vi "Teleop.vi"(10 "Match Info":T1={"Autonomous Elapsed Seconds"=0.0, "TeleOp Elapsed Seconds"=0.0, "Disabled Elapsed Seconds"=0.0, "Visited Autonomous"=FALSE, "Visited TeleOp"=FALSE, "Visited Disabled"=FALSE, "Autonomous Settings"={"Autonomous Style"=enum."Independent", "VI Refnum"=refnum}}, 11 "Call Context":T2) -> ()   [LabVIEW 2016]
doc: "This VI is called for each TeleOp packet received from the DS where the robot is not disabled. It is often used to read from the joysticks and update I/O or to update setpoints for timed control loops. It should complete and return within 20 milliseconds or it may miss DS packets."
uses:
  <vilib>/Rock Robotics/WPI/DriverStation/WPI_DriverStationDerivedRobotMode.ctl
  <vilib>/Rock Robotics/WPI/DriverStation/WPI_DriverStationMatch Info.ctl
  <vilib>/Rock Robotics/WPI/Utilities/WPI_GetSetVariantRefNum.vi
  Robot Global Data.vi
  <vilib>/Rock Robotics/Network Tables/NT Write Boolean Array.vi
  <vilib>/Rock Robotics/Network Tables/NT Write Numeric Array.vi
  <vilib>/Rock Robotics/Network Tables/NT Read Boolean.vi
  <vilib>/Rock Robotics/Network Tables/NT Read Number.vi
  <vilib>/Rock Robotics/WPI/Ultrasonic/WPI_SonarMB1010AnalogRefNum Registry Get.vi
  <vilib>/Rock Robotics/WPI/Ultrasonic/WPI_SonarMB1010AnalogGetRange.vi
  <vilib>/Rock Robotics/Network Tables/NT Write Boolean.vi
  <vilib>/Rock Robotics/Network Tables/NT Write Number.vi
  <vilib>/Rock Robotics/WPI/RobotDrive/WPI_RobotDriveMecanumDrive_Cartesian.vi
panel:
  out "Sample Slider 0":dbl(slide) scale=0.0..5.0
  out "Sample Boolean 1":bool
  out "Sample Boolean 0":bool
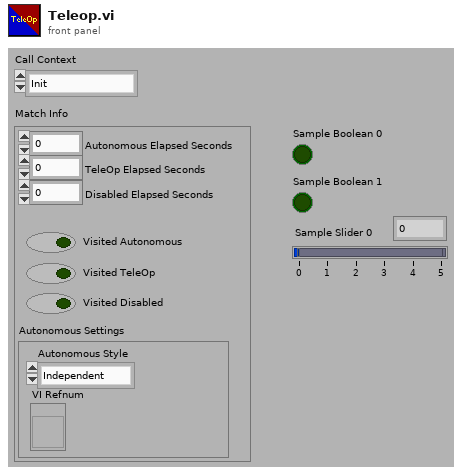
[diagram p1: front panel]
types:
  T1 = typedef "WPI_DriverStationMatch Info.ctl" = cluster{"Autonomous Elapsed Seconds":dbl, "TeleOp Elapsed Seconds":dbl, "Disabled Elapsed Seconds":dbl, "Visited Autonomous":bool, "Visited TeleOp":bool, "Visited Disabled":bool, "Autonomous Settings":cluster{"Autonomous Style":enum16{"Iterative", "Independent"}, "VI Refnum":refnum<vi>}}
  T2 = typedef "WPI_DriverStationDerivedRobotMode.ctl" = enum16{"Init", "Execute", "Stop"}
  T3 = typedef "WPI_JoystickDevRef.ctl" = cluster{"Device":T4}
  T4 = typedef "WPI_JoystickDeviceEnum.ctl" = enum16{"USB 0", "USB 1", "USB 2", "USB 3", "USB 4", "USB 5"}
  T5 = typedef "WPI_RobotDriveDevRef.ctl" = cluster{"DevStatus":errorcluster, "Motors[]":T6[], "Square Inputs":bool, "Max Output":dbl}
  T6 = typedef "WPI_MotorControlDeviceRef.ctl" = cluster{"DeviceStatus":errorcluster, "Type":T7, "PWM":cluster{"PWM Channel":T8, "DeadBand":T9}, "CAN":cluster{"Device Number":u8, "SetOutput VI Ref":variant, "GetOutput VI Ref":variant, "Enable VI Ref":variant, "Disable VI Ref":variant, "Data":variant}, "Invert":bool}
  T7 = typedef "WPI_MotorControlType.ctl" = enum16{"PWM", "CAN"}
  T8 = typedef "FPGA_DIOPWMChannel.ctl" = enum8{"PWM 0", "PWM 1", "PWM 2", "PWM 3", "PWM 4", "PWM 5", "PWM 6", "PWM 7", "PWM 8", "PWM 9", "PWM MXP 0", "PWM MXP 1", "PWM MXP 2", "PWM MXP 3", "PWM MXP 4", "PWM MXP 5", "PWM MXP 6", "PWM MXP 7", "PWM MXP 8", "PWM MXP 9", "Invalid"}
  T9 = typedef "WPI_PWMDeadband.ctl" = cluster{"Name":string, "maxPositivePwm":i32, "minPositivePwm":i32, "centerPwm":i32, "maxNegativePwm":i32, "minNegativePwm":i32, "angularRange":u16}
  T10 = typedef "WPI_ServoDeviceRef.ctl" = cluster{"DeviceStatus":errorcluster, "PWM Channel":T8, "DeadBand":T9}
  T11 = cluster{"Buttons[0]":bool, "Buttons[1]":bool, "Buttons[2]":bool, "Buttons[3]":bool, "Buttons[4]":bool, "Buttons[5]":bool, "Buttons[6]":bool, "Buttons[7]":bool, "Buttons[8]":bool}
  T12 = typedef "WPI_SwitchDevRef.ctl" = cluster{"DevStatus":errorcluster, "DIO Channel":T13, "CntIndex":T14, "Normally Closed":bool}
  T13 = typedef "FPGA_DIOChannel.ctl" = enum8{"DIO 0", "DIO 1", "DIO 2", "DIO 3", "DIO 4", "DIO 5", "DIO 6", "DIO 7", "DIO 8", "DIO 9", "DIO MXP 0", "DIO MXP 1", "DIO MXP 2", "DIO MXP 3", "DIO MXP 4", "DIO MXP 5", "DIO MXP 6", "DIO MXP 7", "DIO MXP 8", "DIO MXP 9", "DIO MXP 10", "DIO MXP 11", "DIO MXP 12", "DIO MXP 13", "DIO MXP 14", "DIO MXP 15", "SPI Port CS1", "SPI Port CS2", "SPI Port CS3", "SPI Port MISO", "SPI Port MOSI", "Invalid"}
  T14 = typedef "FPGA_CounterCtrSystemIndex.ctl" = enum8{"Ctr 0", "Ctr 1", "Ctr 2", "Ctr 3", "Ctr 4", "Ctr 5", "Ctr 6", "Ctr 7", "Invalid"}
  T15 = typedef "WPI_SonarMB1010AnalogDeviceRef.ctl" = cluster{"AIDeviceRef":T16, "Scaling factor (V/in)":dbl, "Average Bits":u8}
  T16 = typedef "WPI_AnalogChannelDevRef.ctl" = cluster{"DevStatus":errorcluster, "Analog Channel":T17}
  T17 = typedef "FPGA_AIChannel.ctl" = enum8{"AI 0", "AI 1", "AI 2", "AI 3", "AI MXP 0", "AI MXP 1", "AI MXP 2", "AI MXP 3", "Invalid"}
  T18 = typedef "WPI_DigitalInputDevRef.ctl" = cluster{"DevStatus":errorcluster, "DIO Channel":T13}
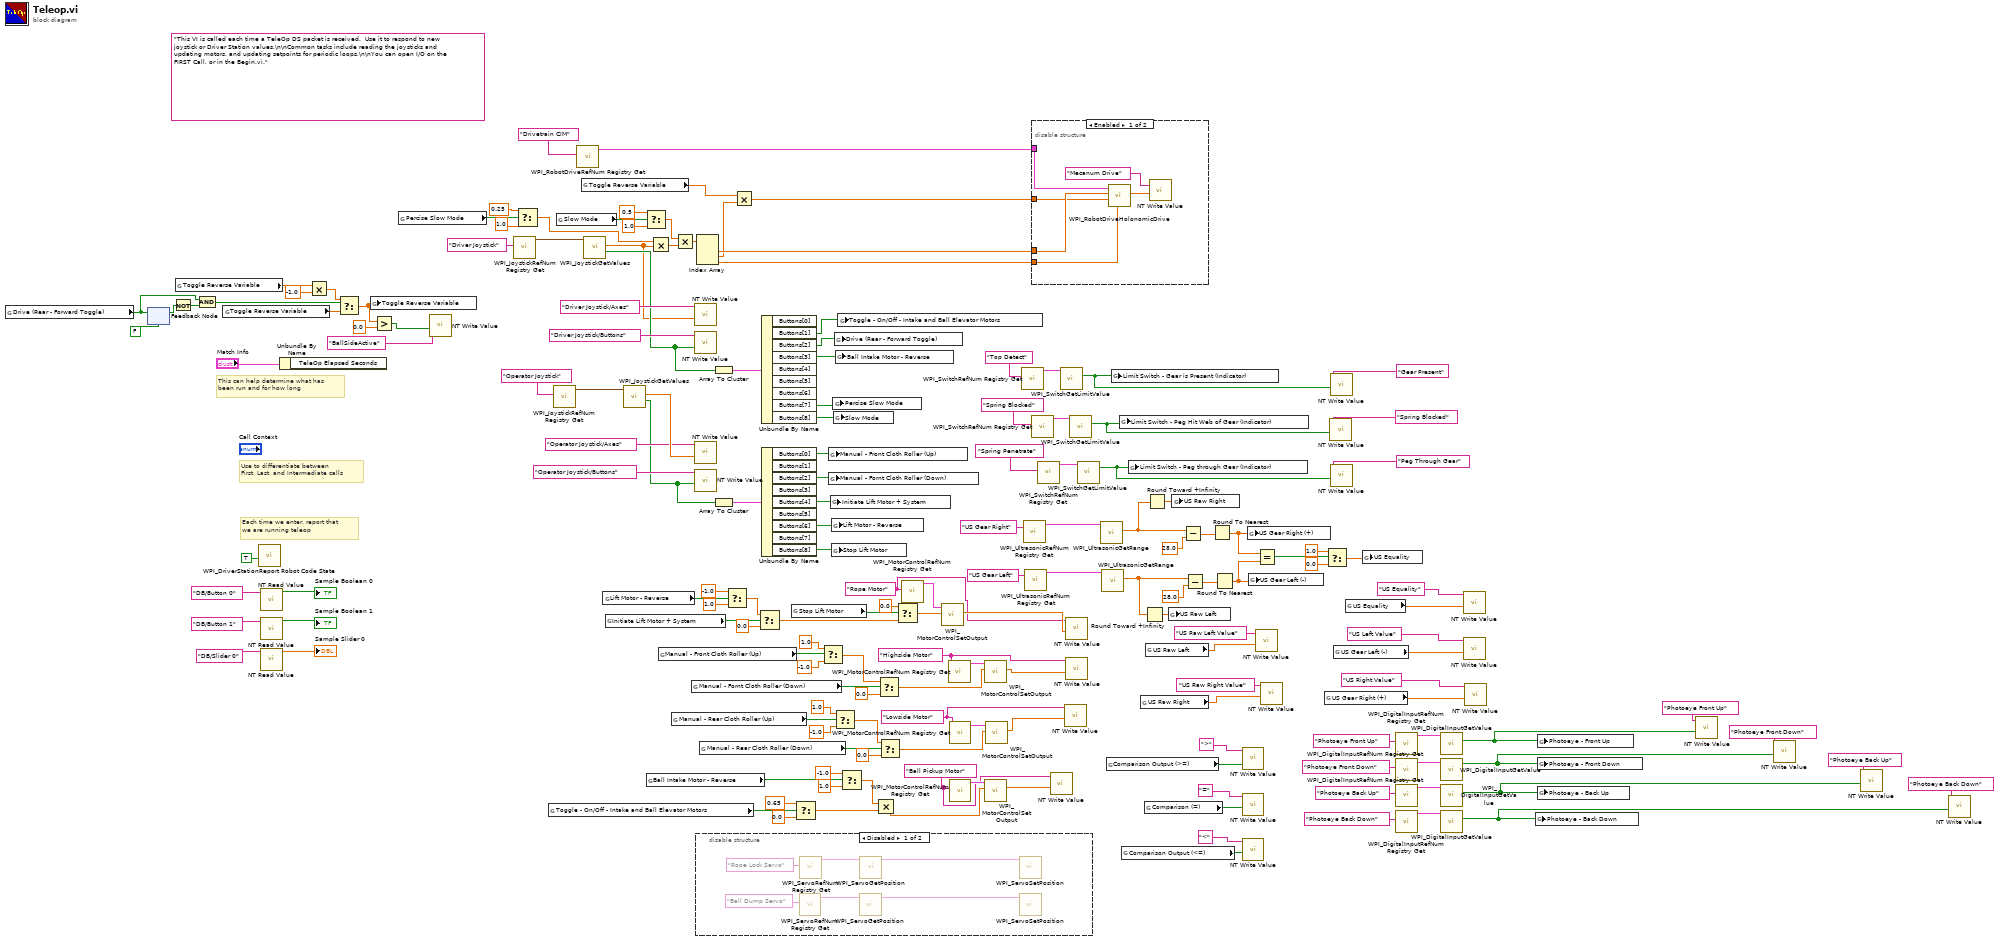
[diagram p0: block diagram]
diagram:
  w5 = "Ball Pickup Motor" ("refnum name")
  w6 = "Lowside Motor" ("refnum name")
  w7 = "Highside Motor" ("refnum name")
  w11 = "Rope Motor" ("refnum name")
  (unwired) "This VI is called each time a TeleOp DS packet is received.  Use it to respond to new joystick or Driver Station values.\n\nCommon tasks include reading the joysticks and updating motors, and updating setpoints for periodic loops.\n\nYou can open I/O on the FIRST Call, or in the Begin.vi."
  # "Each time we enter, report that\nwe are running teleop"
  # "Use to differentiate between\nFirst, Last, and Intermediate calls"
  # "This can help determine what has\nbeen run and for how long"
  n1 = global read "Robot Global Data.vi" "Drive (Rear - Forward Toggle)"() -> (w25:bool)
  n2 = feedback #1(FALSE ("Comparison Output (<=)")) -> (w27:bool)
  n3 = feedback-in #1(w25) -> ()
  n4 = Not(x=w27) -> (.not. x?=w26:bool)
  n5 = global read "Robot Global Data.vi" "Toggle Reverse Variable"() -> (w22:dbl)
  n6 = And(x=w25, y=w26) -> (x .and. y?=w24:bool)
  n7 = global read "Robot Global Data.vi" "Toggle Reverse Variable"() -> (w23:dbl)
  n8 = call <vilib>:"WPI_DriverStationReport Robot Code State.vi"("TeleOp"=TRUE ("Autonomous")) -> ()  [unwired: 10 in, 1 out]
  n9 = call-poly <vilib>:"NT Read Value.vi"("Name"="DB/Button 0" ("refnum name")) -> ("Boolean"=→"Sample Boolean 0":bool)  [unwired: 9 in, 1 out]
  n10 = call-poly <vilib>:"NT Read Value.vi"("Name"="DB/Button 1" ("refnum name")) -> ("Boolean"=→"Sample Boolean 1":bool)  [unwired: 9 in, 1 out]
  n11 = call-poly <vilib>:"NT Read Value.vi"("Name"="DB/Slider 0" ("refnum name")) -> ("Numeric"=→"Sample Slider 0":dbl)  [unwired: 9 in, 1 out]
  n12 = Unbundle By Name("Match Info") -> ()  [unwired: 1 out]
  n13 = Multiply(x=w22, y=-1.0) -> (x*y=w20:dbl)
  n14 = Select(t=w20, s=w24, f=w23) -> (s? t:f=w4:dbl)
  n15 = global write "Robot Global Data.vi" "Toggle Reverse Variable"(w4) -> ()
  n16 = Greater?(x=w4, y=0.0) -> (0:w2:bool)
  n17 = global read "Robot Global Data.vi" "Percise Slow Mode"() -> (w72:bool)
  n18 = call-poly <vilib>:"NT Write Value.vi"("Boolean"=w2, "Name"="BallSideActive") -> ()  [unwired: 9 in, 1 out]
  n19 = call <vilib>:"WPI_JoystickRefNum Registry Get.vi"("refnum name"="Driver Joystick") -> ("JoystickDevRef"=w165:T3)  [unwired: 1 in, 9 out]
  n20 = Select(t=0.25, s=w72, f=1.0) -> (s? t:f=w73:dbl)
  n21 = global read "Robot Global Data.vi" "Toggle - On/Off - Intake and Ball Elevator Motors"() -> (w80:bool)
  n22 = call <vilib>:"WPI_JoystickRefNum Registry Get.vi"("refnum name"="Operator Joystick") -> ("JoystickDevRef"=w147:T3)  [unwired: 9 in, 1 out]
  n23 = global read "Robot Global Data.vi" "Slow Mode"() -> (w151:bool)
  n24 = call <vilib>:"WPI_RobotDriveRefNum Registry Get.vi"("refnum name"="Drivetrain CIM") -> ("RobotDriveDevRef"=w167:T5)  [unwired: 1 in, 9 out]
  n25 = global read "Robot Global Data.vi" "Toggle Reverse Variable"() -> (w17:dbl)
  n26 = call <vilib>:"WPI_JoystickGetValues.vi"("JoystickDevRef"=w165) -> ("Buttons"=w150:bool[], "Axes"=w75:dbl[])  [unwired: 6 in, 3 out]
  n27 = global read "Robot Global Data.vi" "Lift Motor - Reverse"() -> (w103:bool)
  n28 = global read "Robot Global Data.vi" "Initiate Lift Motor + System"() -> (w104:bool)
  n29 = call <vilib>:"WPI_JoystickGetValues.vi"("JoystickDevRef"=w147) -> ("Buttons"=w143:bool[], "Axes"=w146:dbl[])  [unwired: 6 in, 3 out]
  n30 = Select(t=0.5, s=w151, f=1.0) -> (s? t:f=w154:dbl)
  n31 = global read "Robot Global Data.vi" "Ball Intake Motor - Reverse"() -> (w81:bool)
  n32 = Multiply(x=w73, y=w75) -> (x*y=w74:dbl[])
  n33 = global read "Robot Global Data.vi" "Manual - Front Cloth Roller (Up)"() -> (w97:bool)
  n34 = global read "Robot Global Data.vi" "Manual - Rear Cloth Roller (Up)"() -> (w91:bool)
  n35 = Multiply(x=w154, y=w74) -> (x*y=w142:dbl[])
  n36 = global read "Robot Global Data.vi" "Manual - Fornt Cloth Roller (Down)"() -> (w98:bool)
  n37 = call-poly <vilib>:"NT Write Value.vi"("Numeric Array"=w75, "Name"="Driver Joystick/Axes") -> ()  [unwired: 9 in, 1 out]
  n38 = call-poly <vilib>:"NT Write Value.vi"("Boolean Array"=w150, "Name"="Driver Joystick/Buttons") -> ()  [unwired: 9 in, 1 out]
  n39 = call-poly <vilib>:"NT Write Value.vi"("Numeric Array"=w146, "Name"="Operator Joystick/Axes") -> ()  [unwired: 9 in, 1 out]
  n40 = call-poly <vilib>:"NT Write Value.vi"("Boolean Array"=w143, "Name"="Operator Joystick/Buttons") -> ()  [unwired: 9 in, 1 out]
  n41 = disable-structure shown="Disabled" {
    frame Disabled {
      n42 = call <vilib>:"WPI_ServoRefNum Registry Get.vi"("refnum name"="Ball Dump Servo") -> ("ServoDeviceRef"=w173:T10)  [unwired: 9 in, 1 out]
      n43 = call <vilib>:"WPI_ServoRefNum Registry Get.vi"("refnum name"="Rope Lock Servo") -> ("ServoDeviceRef"=w171:T10)  [unwired: 9 in, 1 out]
      n44 = call <vilib>:"WPI_ServoGetPosition.vi"("ServoDeviceRef"=w173) -> ("ServoDeviceRef"=w174:T10)  [unwired: 8 in, 2 out]
      n45 = call <vilib>:"WPI_ServoGetPosition.vi"("ServoDeviceRef"=w171) -> ("ServoDeviceRef"=w172:T10)  [unwired: 8 in, 2 out]
      n46 = call <vilib>:"WPI_ServoSetPosition.vi"("ServoDeviceRef"=w172) -> ()  [unwired: 9 in, 2 out]
      n47 = call <vilib>:"WPI_ServoSetPosition.vi"("ServoDeviceRef"=w174) -> ()  [unwired: 9 in, 2 out]
    }
    frame Enabled {
    }
  }
  n48 = Index Array(array=w142) -> (element #1=w76:dbl, element #2=w19:dbl, element #3=w163:dbl)  [unwired: 3 in]
  n49 = global read "Robot Global Data.vi" "Manual - Rear Cloth Roller (Down)"() -> (w92:bool)
  n50 = Array To Cluster(array=w150) -> (cluster=w149:T11)
  n51 = Array To Cluster(array=w143) -> (cluster=w141:T11)
  n52 = Select(t=-1.0, s=w103, f=1.0) -> (s? t:f=w100:dbl)
  n53 = Multiply(x=w17, y=w19) -> (x*y=w18:dbl)
  n54 = Select(t=w100, s=w104, f=0.0) -> (s? t:f=w54:dbl)
  n55 = Unbundle By Name(w149) -> ("Buttons[1]"=w29:bool, "Buttons[2]"=w31:bool, "Buttons[3]"=w30:bool, "Buttons[7]"=w50:bool, "Buttons[8]"=w49:bool)  [unwired: 4 out]
  n56 = Unbundle By Name(w141) -> ("Buttons[0]"=w140:bool, "Buttons[2]"=w139:bool, "Buttons[4]"=w108:bool, "Buttons[6]"=w107:bool, "Buttons[8]"=w106:bool)  [unwired: 4 out]
  n57 = global read "Robot Global Data.vi" "Stop Lift Motor"() -> (w53:bool)
  n58 = Select(t=0.65, s=w80, f=0.0) -> (s? t:f=w15:dbl)
  n59 = Select(t=1.0, s=w97, f=-1.0) -> (s? t:f=w86:dbl)
  n60 = global write "Robot Global Data.vi" "Manual - Front Cloth Roller (Up)"(w140) -> ()
  n61 = global write "Robot Global Data.vi" "Manual - Fornt Cloth Roller (Down)"(w139) -> ()
  n62 = global write "Robot Global Data.vi" "Initiate Lift Motor + System"(w108) -> ()
  n63 = global write "Robot Global Data.vi" "Lift Motor - Reverse"(w107) -> ()
  n64 = global write "Robot Global Data.vi" "Stop Lift Motor"(w106) -> ()
  n65 = global write "Robot Global Data.vi" "Percise Slow Mode"(w50) -> ()
  n66 = global write "Robot Global Data.vi" "Slow Mode"(w49) -> ()
  n67 = global write "Robot Global Data.vi" "Drive (Rear - Forward Toggle)"(w31) -> ()
  n68 = Select(t=1.0, s=w91, f=-1.0) -> (s? t:f=w84:dbl)
  n69 = global write "Robot Global Data.vi" "Ball Intake Motor - Reverse"(w30) -> ()
  n70 = global write "Robot Global Data.vi" "Toggle - On/Off - Intake and Ball Elevator Motors"(w29) -> ()
  n71 = Select(t=-1.0, s=w81, f=1.0) -> (s? t:f=w14:dbl)
  n72 = Multiply(x=w14, y=w15) -> (x*y=w13:dbl)
  n73 = Select(t=w86, s=w98, f=0.0) -> (s? t:f=w93:dbl)
  n74 = Select(t=w84, s=w92, f=0.0) -> (s? t:f=w87:dbl)
  n75 = Select(t=0.0, s=w53, f=w54) -> (s? t:f=w52:dbl)
  n76 = call <vilib>:"WPI_MotorControlRefNum Registry Get.vi"("refnum name"=w11) -> ("MotorControlDevRef"=w105:T6)  [unwired: 9 in, 1 out]
  n77 = call <vilib>:"WPI_MotorControlSetOutput.vi"("Output"=w52, "MotorControlDevRef"=w105) -> ("Motor Output"=w12:dbl)  [unwired: 7 in, 2 out]
  n78 = call <vilib>:"WPI_MotorControlRefNum Registry Get.vi"("refnum name"=w7) -> ("MotorControlDevRef"=w94:T6)  [unwired: 9 in, 1 out]
  n79 = call <vilib>:"WPI_MotorControlRefNum Registry Get.vi"("refnum name"=w6) -> ("MotorControlDevRef"=w88:T6)  [unwired: 9 in, 1 out]
  n80 = call <vilib>:"WPI_MotorControlRefNum Registry Get.vi"("refnum name"=w5) -> ("MotorControlDevRef"=w82:T6)  [unwired: 9 in, 1 out]
  n81 = call <vilib>:"WPI_MotorControlSetOutput.vi"("Output"=w93, "MotorControlDevRef"=w94) -> ("Motor Output"=w8:dbl)  [unwired: 7 in, 2 out]
  n82 = call <vilib>:"WPI_MotorControlSetOutput.vi"("Output"=w13, "MotorControlDevRef"=w82) -> ("Motor Output"=w10:dbl)  [unwired: 7 in, 2 out]
  n83 = call <vilib>:"WPI_MotorControlSetOutput.vi"("Output"=w87, "MotorControlDevRef"=w88) -> ("Motor Output"=w9:dbl)  [unwired: 7 in, 2 out]
  n84 = call <vilib>:"WPI_SwitchRefNum Registry Get.vi"("refnum name"="Top Detect") -> ("SwitchDevRef"=w137:T12)  [unwired: 9 in, 1 out]
  n85 = call-poly <vilib>:"WPI_UltrasonicRefNum Registry Get.vi"("refnum name"="US Gear Right") -> ("SonarMB1010AnalogDevRef"=w131:T15)  [unwired: 9 in, 1 out]
  n86 = call-poly <vilib>:"WPI_UltrasonicRefNum Registry Get.vi"("refnum name"="US Gear Left") -> ("SonarMB1010AnalogDevRef"=w129:T15)  [unwired: 9 in, 1 out]
  n87 = disable-structure shown="Enabled" {
    disable-tunnel: w167 -> [w181 _]
    disable-tunnel: w163 -> [w180 _]
    disable-tunnel: w76 -> [w177 _]
    disable-tunnel: w18 -> [w176 _]
    frame Enabled {
      n88 = call-poly <vilib>:"WPI_RobotDriveHolonomicDrive.vi"("Rotation"=w180, "Y"=w176, "X"=w177, "RobotDriveDevRef"=w181) -> ("Motor Values"=w178:dbl[])  [unwired: 5 in, 2 out]
      n89 = call-poly <vilib>:"NT Write Value.vi"("Numeric Array"=w178, "Name"="Mecanum Drive") -> ()  [unwired: 9 in, 1 out]
    }
    frame Disabled {
    }
  }
  n90 = call <vilib>:"WPI_SwitchRefNum Registry Get.vi"("refnum name"="Spring Blocked") -> ("SwitchDevRef"=w135:T12)  [unwired: 9 in, 1 out]
  n91 = call <vilib>:"WPI_SwitchRefNum Registry Get.vi"("refnum name"="Spring Penetrate") -> ("SwitchDevRef"=w134:T12)  [unwired: 9 in, 1 out]
  n92 = call-poly <vilib>:"NT Write Value.vi"("Numeric"=w10, "Name"=w5) -> ()  [unwired: 9 in, 1 out]
  n93 = call <vilib>:"WPI_SwitchGetLimitValue.vi"("SwitchDevRef"=w137) -> ("Switch Pressed"=w69:bool)  [unwired: 8 in, 2 out]
  n94 = call-poly <vilib>:"NT Write Value.vi"("Numeric"=w9, "Name"=w6) -> ()  [unwired: 9 in, 1 out]
  n95 = call-poly <vilib>:"NT Write Value.vi"("Numeric"=w12, "Name"=w11) -> ()  [unwired: 9 in, 1 out]
  n96 = call-poly <vilib>:"NT Write Value.vi"("Numeric"=w8, "Name"=w7) -> ()  [unwired: 9 in, 1 out]
  n97 = call <vilib>:"WPI_SwitchGetLimitValue.vi"("SwitchDevRef"=w135) -> ("Switch Pressed"=w111:bool)  [unwired: 8 in, 2 out]
  n98 = call <vilib>:"WPI_SwitchGetLimitValue.vi"("SwitchDevRef"=w134) -> ("Switch Pressed"=w67:bool)  [unwired: 8 in, 2 out]
  n99 = call-poly <vilib>:"WPI_UltrasonicGetRange.vi"("SonarMB1010AnalogDevRef"=w131) -> ("Distance"=w57:dbl)  [unwired: 8 in, 2 out]
  n100 = call-poly <vilib>:"WPI_UltrasonicGetRange.vi"("SonarMB1010AnalogDevRef"=w129) -> ("Distance"=w59:dbl)  [unwired: 8 in, 2 out]
  n101 = global read "Robot Global Data.vi" "Comparison Output (>=)"() -> (w63:bool)
  n102 = global write "Robot Global Data.vi" "Limit Switch - Gear is Present (Indicator)"(w69) -> ()
  n103 = global write "Robot Global Data.vi" "Limit Switch - Peg Hit Web of Gear (Indicator)"(w111) -> ()
  n104 = global read "Robot Global Data.vi" "Comparison Output (<=)"() -> (w64:bool)
  n105 = global write "Robot Global Data.vi" "Limit Switch - Peg through Gear (Indicator)"(w67) -> ()
  n106 = global read "Robot Global Data.vi" "US Raw Right"() -> (w55:dbl)
  n107 = Round Toward +Infinity(x=w59) -> (ceil(x): smallest int >= x=w32:dbl)
  n108 = global read "Robot Global Data.vi" "Comparison (=)"() -> (w65:bool)
  n109 = global read "Robot Global Data.vi" "US Raw Left"() -> (w56:dbl)
  n110 = Round Toward +Infinity(x=w57) -> (ceil(x): smallest int >= x=w58:dbl)
  n111 = global write "Robot Global Data.vi" "US Raw Left"(w32) -> ()
  n112 = global write "Robot Global Data.vi" "US Raw Right"(w58) -> ()
  n113 = Subtract(x=w57, y=28.0) -> (x-y=w121:dbl)
  n114 = Subtract(x=w59, y=28.0) -> (x-y=w122:dbl)
  n115 = Round To Nearest(number=w121) -> (nearest integer value=w120:dbl)
  n116 = Round To Nearest(number=w122) -> (nearest integer value=w119:dbl)
  n117 = call-poly <vilib>:"NT Write Value.vi"("Boolean"=w63, "Name"=">") -> ()  [unwired: 9 in, 1 out]
  n118 = call-poly <vilib>:"NT Write Value.vi"("Boolean"=w65, "Name"="=") -> ()  [unwired: 9 in, 1 out]
  n119 = call-poly <vilib>:"NT Write Value.vi"("Boolean"=w64, "Name"="<") -> ()  [unwired: 9 in, 1 out]
  n120 = global write "Robot Global Data.vi" "US Gear Right (+)"(w120) -> ()
  n121 = global write "Robot Global Data.vi" "US Gear Left (-)"(w119) -> ()
  n122 = call-poly <vilib>:"NT Write Value.vi"("Numeric"=w56, "Name"="US Raw Left Value") -> ()  [unwired: 9 in, 1 out]
  n123 = Equal?(x=w120, y=w119) -> (x = y?=w118:bool)
  n124 = call-poly <vilib>:"NT Write Value.vi"("Numeric"=w55, "Name"="US Raw Right Value") -> ()  [unwired: 9 in, 1 out]
  n125 = global read "Robot Global Data.vi" "US Gear Right (+)"() -> (w127:dbl)
  n126 = Select(t=1.0, s=w118, f=0.0) -> (s? t:f=w117:dbl)
  n127 = call-poly <vilib>:"NT Write Value.vi"("Boolean"=w111, "Name"="Spring Blocked") -> ()  [unwired: 9 in, 1 out]
  n128 = call-poly <vilib>:"NT Write Value.vi"("Boolean"=w69, "Name"="Gear Present") -> ()  [unwired: 9 in, 1 out]
  n129 = call-poly <vilib>:"NT Write Value.vi"("Boolean"=w67, "Name"="Peg Through Gear") -> ()  [unwired: 9 in, 1 out]
  n130 = global read "Robot Global Data.vi" "US Gear Left (-)"() -> (w125:dbl)
  n131 = global read "Robot Global Data.vi" "US Equality"() -> (w116:dbl)
  n132 = global write "Robot Global Data.vi" "US Equality"(w117) -> ()
  n133 = call <vilib>:"WPI_DigitalInputRefNum Registry Get.vi"("refnum name"="Photoeye Front Up") -> ("DigitalInputDevRef"=w47:T18)  [unwired: 9 in, 1 out]
  n134 = call <vilib>:"WPI_DigitalInputRefNum Registry Get.vi"("refnum name"="Photoeye Front Down") -> ("DigitalInputDevRef"=w45:T18)  [unwired: 9 in, 1 out]
  n135 = call <vilib>:"WPI_DigitalInputRefNum Registry Get.vi"("refnum name"="Photoeye Back Up") -> ("DigitalInputDevRef"=w41:T18)  [unwired: 9 in, 1 out]
  n136 = call <vilib>:"WPI_DigitalInputRefNum Registry Get.vi"("refnum name"="Photoeye Back Down") -> ("DigitalInputDevRef"=w42:T18)  [unwired: 9 in, 1 out]
  n137 = call <vilib>:"WPI_DigitalInputGetValue.vi"("DigitalInputDevRef"=w47) -> ("Value"=w40:bool)  [unwired: 8 in, 2 out]
  n138 = call <vilib>:"WPI_DigitalInputGetValue.vi"("DigitalInputDevRef"=w45) -> ("Value"=w38:bool)  [unwired: 8 in, 2 out]
  n139 = call <vilib>:"WPI_DigitalInputGetValue.vi"("DigitalInputDevRef"=w41) -> ("Value"=w36:bool)  [unwired: 8 in, 2 out]
  n140 = call <vilib>:"WPI_DigitalInputGetValue.vi"("DigitalInputDevRef"=w42) -> ("Value"=w33:bool)  [unwired: 8 in, 2 out]
  n141 = call-poly <vilib>:"NT Write Value.vi"("Numeric"=w116, "Name"="US Equality") -> ()  [unwired: 9 in, 1 out]
  n142 = call-poly <vilib>:"NT Write Value.vi"("Numeric"=w125, "Name"="US Left Value") -> ()  [unwired: 9 in, 1 out]
  n143 = call-poly <vilib>:"NT Write Value.vi"("Numeric"=w127, "Name"="US Right Value") -> ()  [unwired: 9 in, 1 out]
  n144 = global write "Robot Global Data.vi" "Photoeye - Back Down"(w33) -> ()
  n145 = global write "Robot Global Data.vi" "Photoeye - Front Up"(w40) -> ()
  n146 = global write "Robot Global Data.vi" "Photoeye - Front Down"(w38) -> ()
  n147 = global write "Robot Global Data.vi" "Photoeye - Back Up"(w36) -> ()
  n148 = call-poly <vilib>:"NT Write Value.vi"("Boolean"=w40, "Name"="Photoeye Front Up") -> ()  [unwired: 9 in, 1 out]
  n149 = call-poly <vilib>:"NT Write Value.vi"("Boolean"=w38, "Name"="Photoeye Front Down") -> ()  [unwired: 9 in, 1 out]
  n150 = call-poly <vilib>:"NT Write Value.vi"("Boolean"=w36, "Name"="Photoeye Back Up") -> ()  [unwired: 9 in, 1 out]
  n151 = call-poly <vilib>:"NT Write Value.vi"("Boolean"=w33, "Name"="Photoeye Back Down") -> ()  [unwired: 9 in, 1 out]
